vi "rqcAlice PM Level Test (Low Level Example).vi"() -> ()   [LabVIEW 2018]
uses:
  FPGA/Alice/Custom Controls/Main State Machine/rqcAlice DAC Clock Positions.ctl
  Shared/Shared FPGA Lib/Shared Logic/Custom Controls/rqc Random Generator.parameters.ctl
  Shared/Shared FPGA Lib/Shared Logic/Custom Controls/rqc Random Generator.value type.ctl
  FPGA/Alice/Custom Controls/Phase Modulator/rqcAlice Mod.Config.ctl
  Custom Controls/rqcAlice States.ctl
  Shared/Shared Host Lib/rqc ServiceNET/Custom Controls/rqc ServiceNET command.ctl
  Shared/Shared Host Lib/rqc ServiceNET/Alice/Custom Controls/rqcAlice ServiceNET control.ctl
  <vilib>/FPGAPlugInAG/PCI-7811R/niLvFpga_Open_PCI-7811R.vi
  <vilib>/rvi/interface/common/dynamic/niFpgaDynamicAddResources.vi
  <vilib>/FPGAPlugInAG/Dynamic/niLvFpga_Close_Dynamic.vi
  <vilib>/rvi/interface/nirviOpenFPGA/nirviOpenFPGA.xnode
  FPGA Bitfiles/rqcAlice FPGA (7811R) v 3.0.0.lvbitx
  <vilib>/rvi/interface/nirviCloseFPGA/nirviCloseFPGA.xnode
panel:
  in  "Attenuation, dB":fxp<+,7,6>
  in  "Delay Line":u32=24665
  out "XY Graph":T1(graph)={"appended array"=[0.0, 8.0, 16.0, 24.0, 32.0, 40.0, 48.0, 56.0, 64.0, 72.0, 80.0, 88.0, 96.0, 104.0, 112.0, 120.0, 128.0, 136.0, 144.0, 152.0, 160.0, 168.0, 176.0, 184.0, 192.0, 200.0, 208.0, 216.0, 224.0, 232.0, 240.0, 248.0, 256.0, 264.0, 272.0, 280.0, 288.0, 296.0, 304.0, 312.0, 320.0, 328.0, 336.0, 344.0, 352.0, 360.0, 368.0, 376.0, 384.0, 392.0, 400.0, 408.0, 416.0, 424.0, 432.0, 440.0, 448.0, 456.0, 464.0, 472.0, 480.0, 488.0, 496.0, 504.0, 512.0, 512.0], "appended array"=[4.0, 1.0, 6.0, 11.0, 18.0, 22.0, 32.0, 57.0, 67.0, 85.0, 91.0, 122.0, 128.0, 130.0, 145.0, 171.0, 185.0, 166.0, 196.0, 178.0, 195.0, 205.0, 197.0, 198.0, 189.0, 183.0, 188.0, 184.0, 164.0, 143.0, 127.0, 129.0, 123.0, 108.0, 77.0, 63.0, 51.0, 62.0, 40.0, 26.0, 19.0, 17.0, 19.0, 26.0, 15.0, 21.0, 28.0, 23.0, 40.0, 36.0, 69.0, 61.0, 58.0, 96.0, 93.0, 110.0, 128.0, 93.0, 112.0, 128.0, 125.0, 144.0, 161.0, 159.0, 158.0]}
  out "PM Value":u16=512
  in  "PM Delta":u16=8
  in  "PM max":u16=512
  in  "PM min":u16
  out "error out":errorcluster
  in  "Stop":bool
  out "connected?":bool
  in  "port":u16=5020
  out "Current State":T2=enum."App.Stop"
  in  "Modulator config":T3={"mod.on"=9, "mod.off"=2}
  in  "PM.DAC parameters":T4={"value type"=enum."constant", "constant"=512, "num of levels"=0, "levels values"=[512, 512, 512, 512]}
  in  "DAC Clock positions":T6=[18, 38]
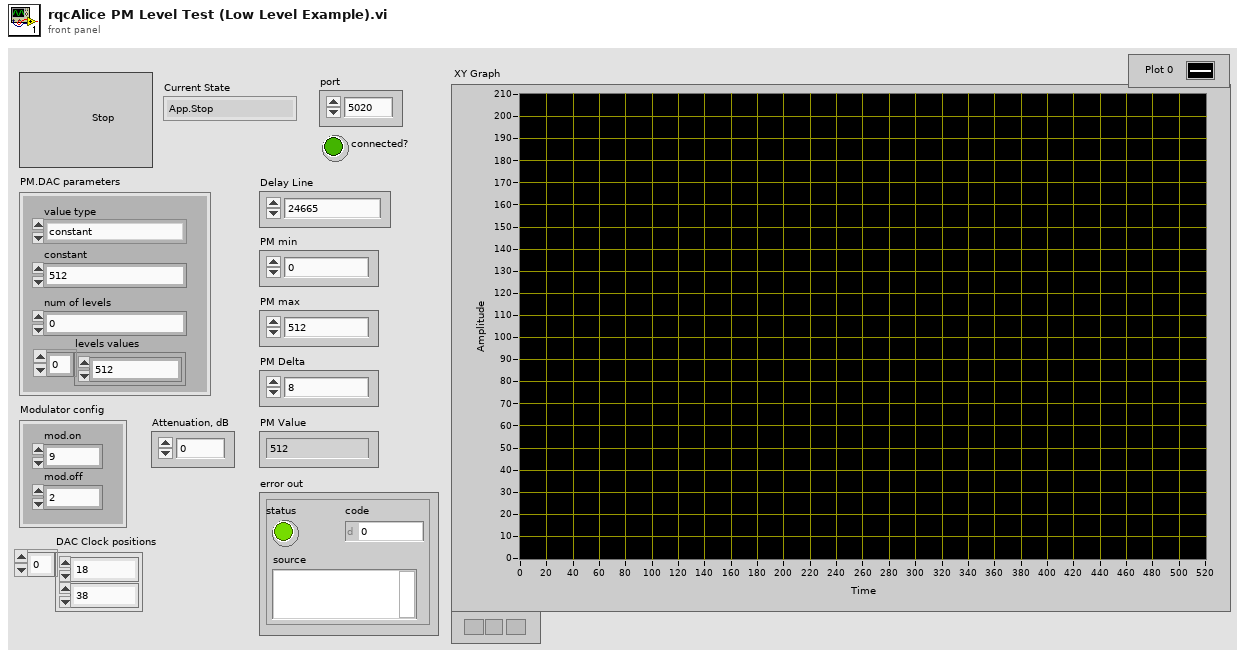
[diagram p1: front panel]
types:
  T1 = cluster{"appended array":dbl[], "appended array":dbl[]}
  T2 = typedef "rqcAlice States.ctl" = enum16{"HW.configure", "HW.meas", "NET.create", "NET.connect", "NET.readCommand", "NET.sendCommand", "NET.readData", "NET.close", "Meas.Start", "Meas.NextStep", "Meas.restart", "Meas.Done", "App.HandleEvent", "App.HandleError", "App.Stop"}
  T3 = typedef "rqcAlice Mod.Config.ctl" = cluster{"mod.on":u8, "mod.off":u8}
  T4 = typedef "rqc Random Generator.parameters.ctl" = cluster{"value type":T5, "constant":u16, "num of levels":u16, "levels values":u16[]}
  T5 = typedef "rqc Random Generator.value type.ctl" = enum16{"random value", "constant"}
  T6 = typedef "rqcAlice DAC Clock Positions.ctl" = u8[]
  T7 = typedef "rqc ServiceNET command.ctl" = enum8{"NONE", "READY", "START", "PING"}
  T8 = typedef "rqcAlice ServiceNET control.ctl" = cluster{"connection ID":refnum<k5>, "port":u16, "connected?":bool}
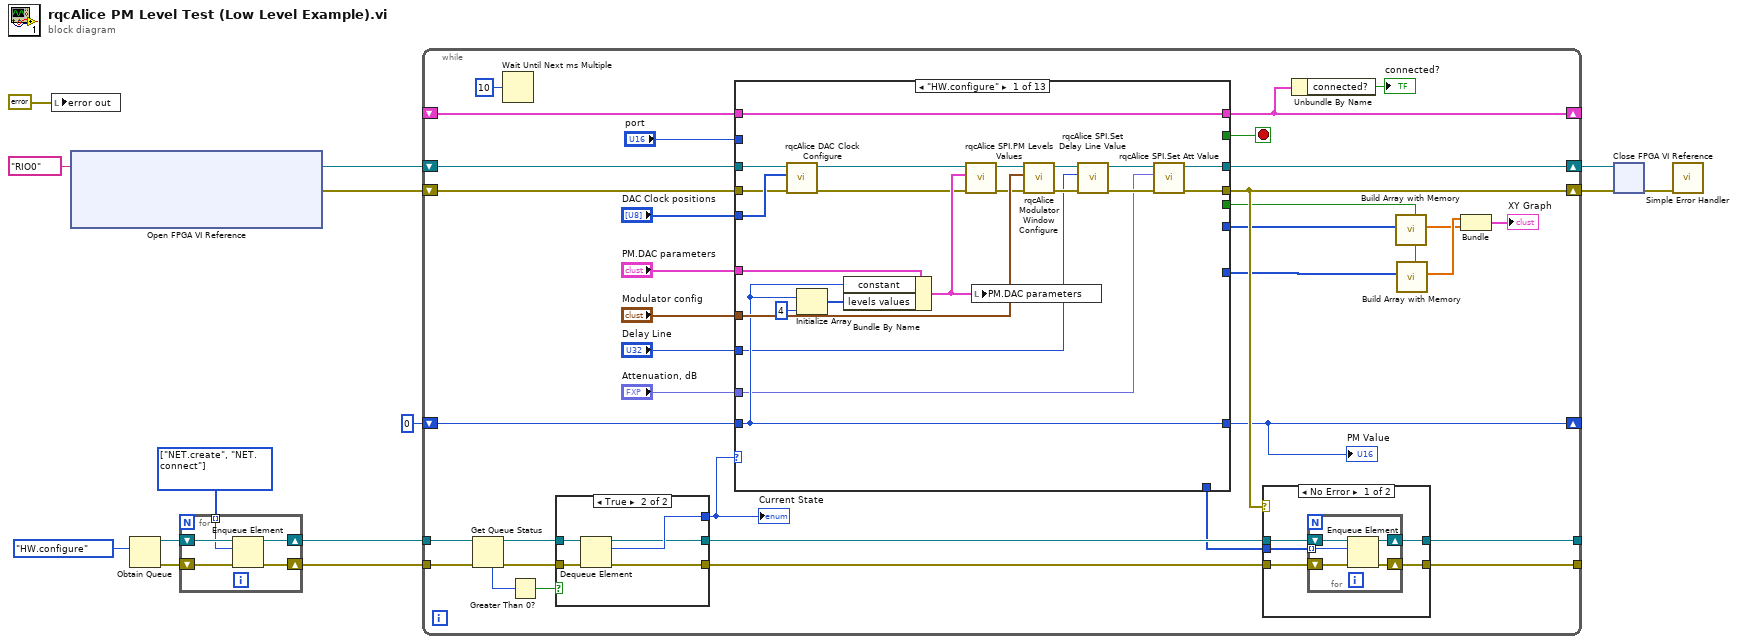
[diagram p0: block diagram]
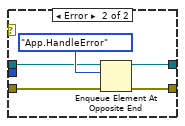
[diagram p2: hidden frame]
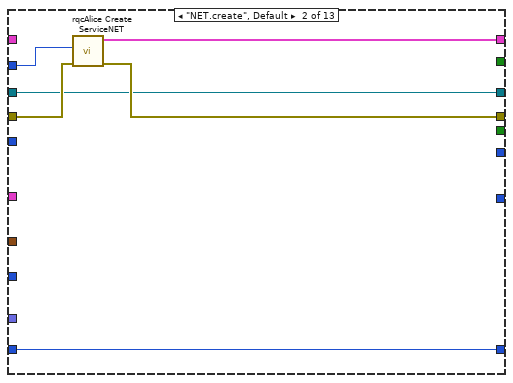
[diagram p3: hidden frame]
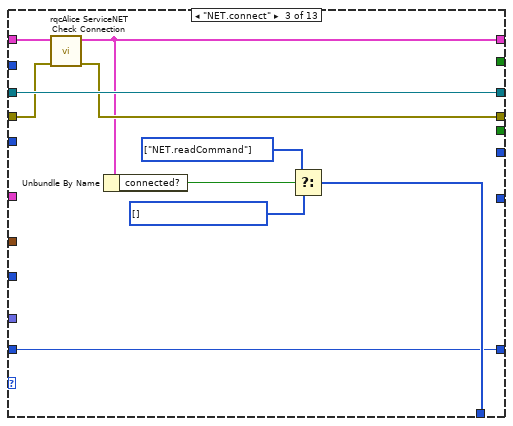
[diagram p4: hidden frame]
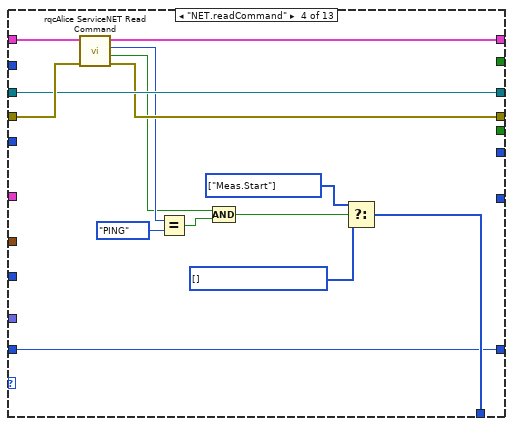
[diagram p5: hidden frame]
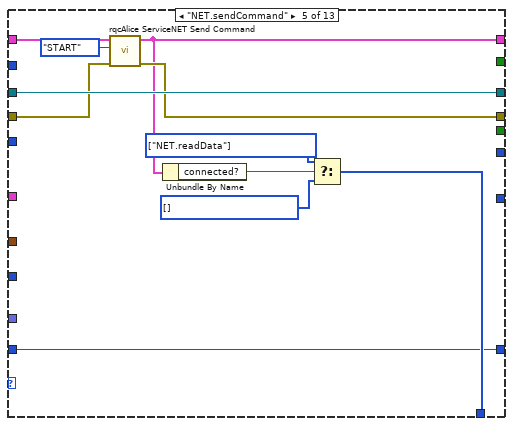
[diagram p6: hidden frame]
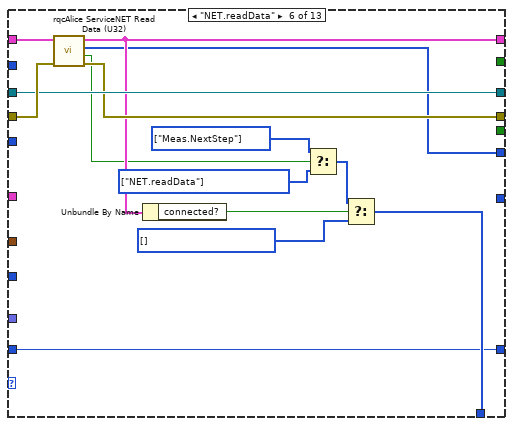
[diagram p7: hidden frame]
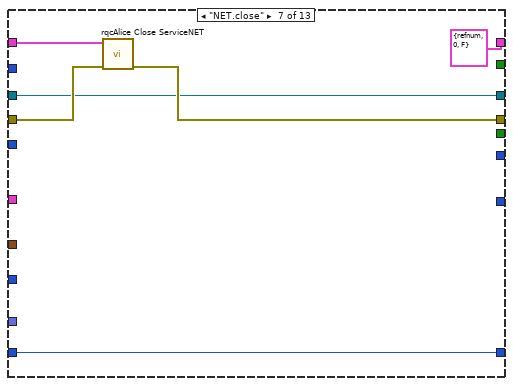
[diagram p8: hidden frame]
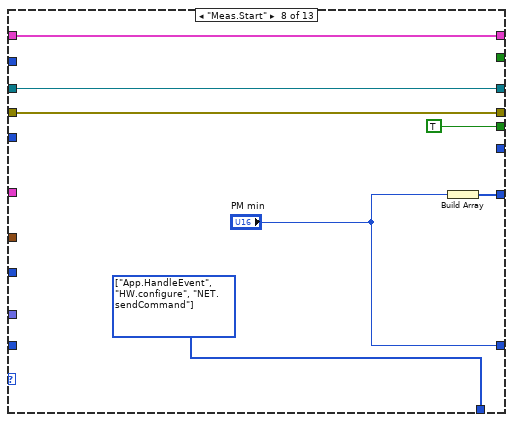
[diagram p9: hidden frame]
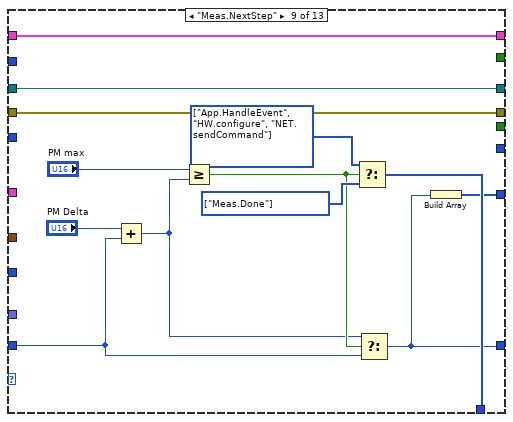
[diagram p10: hidden frame]
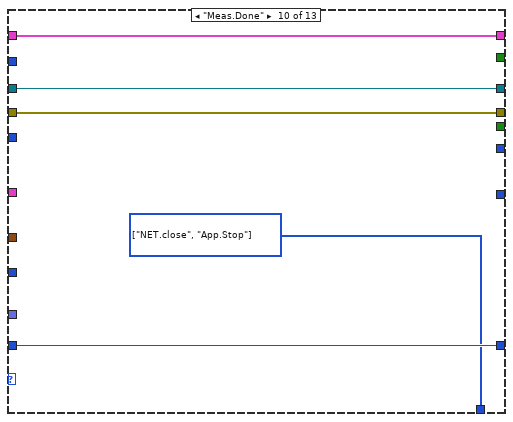
[diagram p11: hidden frame]
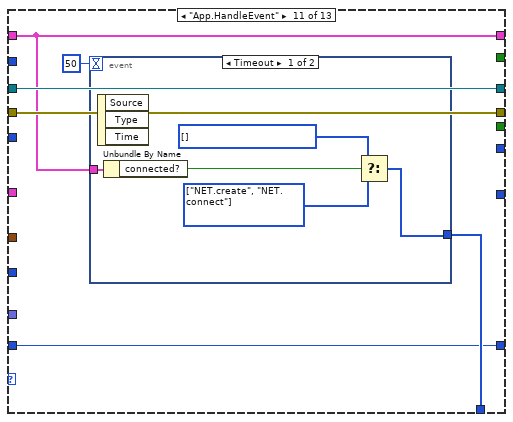
[diagram p12: hidden frame]
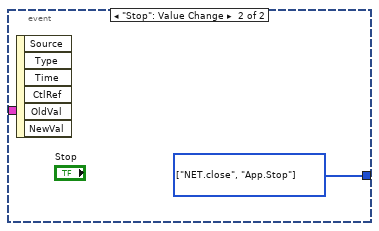
[diagram p13: hidden frame]
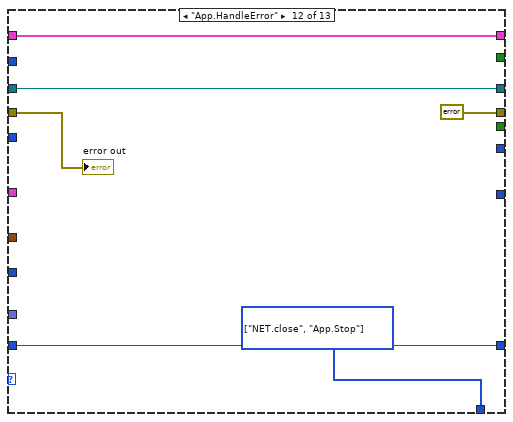
[diagram p14: hidden frame]
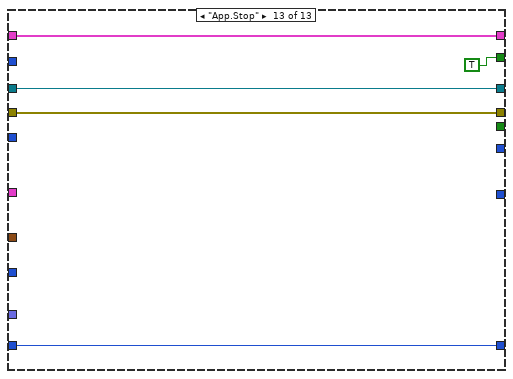
[diagram p15: hidden frame]
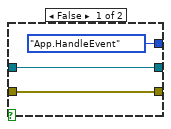
[diagram p16: hidden frame]
diagram:
  w6 = T2[] [enum."NET.create", enum."NET.connect"] items=["HW.configure", "HW.meas", "NET.create", "NET.connect", "NET.readCommand", "NET.sendCommand", "NET.readData", "NET.close", "Meas.Start", "Meas.NextStep", "Meas.restart", "Meas.Done", "App.HandleEvent", "App.HandleError", "App.Stop"]
  n1 = local write "error out"(errorcluster {"status"=FALSE, "code"=0, "source"=""} ("error out")) -> ()
  n2 = xnode "Open FPGA VI Reference"("resource name"=tag "RIO0") -> ("FPGA VI Reference Out"=w13:refnum<k20>, "error out"=w12:errorcluster)  [unwired: 1 in]
  n3 = Obtain Queue(element data type=rqcAlice_States."HW.configure" ("rqcAlice States")) -> (queue out=w8:refnum<queue>, error out=w7:errorcluster)  [unwired: 4 in, 1 out]
  n4 = for {
    shift-right: [w17] -> w5
    shift-left: w8 -> [w19]
    shift-right: [w16] -> w4
    shift-left: w7 -> [w18]
    tunnel: w6 -> [w15] mode=indexing
    n5 = Enqueue Element(queue=w19, element=w15, error in (no error)=w18) -> (queue out=w17:refnum<queue>, error out=w16:errorcluster)  [unwired: 1 in, 1 out]
  }
  n6 = while {
    tunnel: w5 -> [w48]
    shift-right: [w49] -> w11
    shift-left: w13 -> [w54]
    shift-right: [w41] -> w10
    shift-left: w12 -> [w52]
    tunnel: w4 -> [w47]
    tunnel: [w38] -> _
    tunnel: [w37] -> _
    shift-right: [w33] -> _
    shift-left: _ -> [w35]
    shift-right: [w27] -> _
    shift-left: u16 0 ("Delay Line min") -> [w29]
    stop <- w31 stop-if-true
    n7 = Get Queue Status(queue=w48, error in (no error)=w47) -> (queue out=w44:refnum<queue>, error out=w43:errorcluster, # elements in queue=w46:i32)  [unwired: 1 in, 5 out]
    n8 = Wait Until Next ms Multiple(millisecond multiple=u32 10) -> ()  [unwired: 1 out]
    n9 = Greater Than 0?(x=w46) -> (x > 0?=w45:bool)
    n10 = case shown="True" w45 {
      tunnel: w44 -> [w202 w208]
      tunnel: w43 -> [w201 w207]
      tunnel: [rqcAlice_States."App.HandleEvent" ("rqcAlice States") w206] -> w42
      tunnel: [w202 w205] -> w40
      tunnel: [w201 w204] -> w39
      frame False {
      }
      frame True {
        n11 = Dequeue Element(queue=w208, error in (no error)=w207) -> (queue out=w205:refnum<queue>, element=w206:T2, error out=w204:errorcluster)  [unwired: 1 in, 1 out]
      }
    }
    "Current State" <- w42
    n12 = case shown="\"HW.configure\"" w42 {
      tunnel: w54 -> [w91 w94 w107 w118 w132 w144 w148 w158 w171 w176 w183 w194 w199]
      tunnel: "DAC Clock positions" -> [w90 _ _ _ _ _ _ _ _ _ _ _ _]
      tunnel: w52 -> [w89 w96 w105 w120 w130 w145 w151 w157 w170 w175 w182 w193 w198]
      tunnel: "PM.DAC parameters" -> [w86 _ _ _ _ _ _ _ _ _ _ _ _]
      tunnel: "Modulator config" -> [w88 _ _ _ _ _ _ _ _ _ _ _ _]
      tunnel: [w78 w94 w107 w118 w132 w144 w148 w158 w171 w176 w183 w194 w199] -> w49
      tunnel: [w76 w95 w104 w117 w129 w143 w150 w157 w170 w175 w182 errorcluster {"status"=FALSE, "code"=0, "source"=""} ("error out") w198] -> w41
      tunnel: [_ _ w100 w109 w123 w135 _ w156 w166 w173 w179 w191 _] -> w36
      tunnel: [w87 w97 w103 w119 w127 w142 T8 {"connection ID"=refnum, "port"=0, "connected?"=FALSE} ("rqcAlice ServiceNET out") w159 w172 w177 w180 w195 w197] -> w33
      tunnel: w35 -> [w87 _ w106 w121 w131 w146 w152 w159 w172 w177 w180 w195 w197]
      tunnel: "port" -> [_ w93 _ _ _ _ _ _ _ _ _ _ _]
      tunnel: [_ _ _ _ _ _ _ _ _ _ _ _ TRUE] -> w31
      tunnel: w29 -> [w83 w92 w98 w108 w122 w134 w147 _ w162 w174 w178 w190 w196]
      tunnel: [w83 w92 w98 w108 w122 w134 w147 "PM min" w161 w174 w178 w190 w196] -> w27
      tunnel: [_ _ _ _ _ w133 _ _ _ _ _ _ _] -> w28
      tunnel: [_ _ _ _ _ _ _ w153 w160 _ _ _ _] -> w26
      tunnel: [_ _ _ _ _ _ _ TRUE _ _ _ _ _] -> w25
      tunnel: "Delay Line" -> [w80 _ _ _ _ _ _ _ _ _ _ _ _]
      tunnel: "Attenuation, dB" -> [w75 _ _ _ _ _ _ _ _ _ _ _ _]
      frame "HW.configure" {
        n13 = call "rqcAlice DAC Clock Configure.vi"("error in"=w89, "DAC Clock params"=w90, "Alice FPGA Reference In"=w91) -> ("error out"=w72:errorcluster, "Alice FPGA Reference Out"=w74:refnum<k20>)  [unwired: 7 in]
        n14 = Initialize Array(w83, 4 ("dimension size")) -> (w84:u16[])
        n15 = Bundle By Name(cluster=w86, "constant"=w83, "levels values"=w84) -> (w73:T4)
        n16 = call "rqcAlice SPI.PM Levels Values.vi"("error in"=w72, "RndGen.parameters"=w73, "Alice FPGA Reference In"=w74) -> ("error out"=w71:errorcluster, "Alice FPGA Reference Out"=w70:refnum<k20>)  [unwired: 6 in, 1 out]
        n17 = local write "PM.DAC parameters"(w73) -> ()
        n18 = call "rqcAlice Modulator Window Configure.vi"("error in"=w71, "Modulator config"=w88, "Alice FPGA Reference In"=w70) -> ("error out"=w82:errorcluster, "Alice FPGA Reference Out"=w81:refnum<k20>)  [unwired: 7 in]
        n19 = call "rqcAlice SPI.Set Delay Line Value.vi"("error in"=w82, "Delay Line Value"=w80, "Alice FPGA Reference In"=w81) -> ("error out"=w77:errorcluster, "Alice FPGA Reference Out"=w79:refnum<k20>)  [unwired: 7 in]
        n20 = call "rqcAlice SPI.Set Att Value.vi"("error in"=w77, "Attenuation, dB"=w75, "Alice FPGA Reference In"=w79) -> ("error out"=w76:errorcluster, "Alice FPGA Reference Out"=w78:refnum<k20>)  [unwired: 7 in]
      }
      frame "NET.create", Default {
        n21 = call "rqcAlice Create ServiceNET.vi"("error in"=w96, "port"=w93) -> ("error out"=w95:errorcluster, "rqcAlice ServiceNET control"=w97:T8)  [unwired: 8 in]
      }
      frame "NET.connect" {
        w99 = T2[] [] items=["HW.configure", "HW.meas", "NET.create", "NET.connect", "NET.readCommand", "NET.sendCommand", "NET.readData", "NET.close", "Meas.Start", "Meas.NextStep", "Meas.restart", "Meas.Done", "App.HandleEvent", "App.HandleError", "App.Stop"] ("f")
        w101 = T2[] [enum."NET.readCommand"] items=["HW.configure", "HW.meas", "NET.create", "NET.connect", "NET.readCommand", "NET.sendCommand", "NET.readData", "NET.close", "Meas.Start", "Meas.NextStep", "Meas.restart", "Meas.Done", "App.HandleEvent", "App.HandleError", "App.Stop"]
        n22 = call "rqcAlice ServiceNET Check Connection.vi"("error in"=w105, "rqcAlice ServiceNET in"=w106) -> ("error out"=w104:errorcluster, "rqcAlice ServiceNET out"=w103:T8)  [unwired: 8 in]
        n23 = Unbundle By Name(w103) -> ("connected?"=w102:bool)
        n24 = Select(t=w101, s=w102, f=w99) -> (s? t:f=w100:T2[])
      }
      frame "NET.readCommand" {
        w110 = T2[] [] items=["HW.configure", "HW.meas", "NET.create", "NET.connect", "NET.readCommand", "NET.sendCommand", "NET.readData", "NET.close", "Meas.Start", "Meas.NextStep", "Meas.restart", "Meas.Done", "App.HandleEvent", "App.HandleError", "App.Stop"] ("f")
        w111 = T2[] [enum."Meas.Start"] items=["HW.configure", "HW.meas", "NET.create", "NET.connect", "NET.readCommand", "NET.sendCommand", "NET.readData", "NET.close", "Meas.Start", "Meas.NextStep", "Meas.restart", "Meas.Done", "App.HandleEvent", "App.HandleError", "App.Stop"] ("f")
        n25 = call "rqcAlice ServiceNET Read Command.vi"("error in"=w120, "rqcAlice ServiceNET in"=w121) -> ("error out"=w117:errorcluster, "cmd valid"=w113:bool, "command"=w115:T7, "rqcAlice ServiceNET out"=w119:T8)  [unwired: 6 in]
        n26 = Equal?(x=w115, y=rqc_ServiceNET_command."PING" ("command")) -> (x = y?=w114:bool)
        n27 = Compound Arithmetic op=AND(w113, w114) -> (w112:bool)
        n28 = Select(t=w111, s=w112, f=w110) -> (s? t:f=w109:T2[])
      }
      frame "NET.sendCommand" {
        w124 = T2[] [] items=["HW.configure", "HW.meas", "NET.create", "NET.connect", "NET.readCommand", "NET.sendCommand", "NET.readData", "NET.close", "Meas.Start", "Meas.NextStep", "Meas.restart", "Meas.Done", "App.HandleEvent", "App.HandleError", "App.Stop"] ("f")
        w125 = T2[] [enum."NET.readData"] items=["HW.configure", "HW.meas", "NET.create", "NET.connect", "NET.readCommand", "NET.sendCommand", "NET.readData", "NET.close", "Meas.Start", "Meas.NextStep", "Meas.restart", "Meas.Done", "App.HandleEvent", "App.HandleError", "App.Stop"] ("f")
        n29 = call "rqcAlice ServiceNET Send Command.vi"("error in"=w130, "command"=rqc_ServiceNET_command."START", "rqcAlice ServiceNET in"=w131) -> ("error out"=w129:errorcluster, "rqcAlice ServiceNET out"=w127:T8)  [unwired: 7 in]
        n30 = Unbundle By Name(w127) -> ("connected?"=w126:bool)
        n31 = Select(t=w125, s=w126, f=w124) -> (s? t:f=w123:T2[])
      }
      frame "NET.readData" {
        w136 = T2[] [] items=["HW.configure", "HW.meas", "NET.create", "NET.connect", "NET.readCommand", "NET.sendCommand", "NET.readData", "NET.close", "Meas.Start", "Meas.NextStep", "Meas.restart", "Meas.Done", "App.HandleEvent", "App.HandleError", "App.Stop"] ("f")
        w141 = T2[] [enum."Meas.NextStep"] items=["HW.configure", "HW.meas", "NET.create", "NET.connect", "NET.readCommand", "NET.sendCommand", "NET.readData", "NET.close", "Meas.Start", "Meas.NextStep", "Meas.restart", "Meas.Done", "App.HandleEvent", "App.HandleError", "App.Stop"] ("t")
        w139 = T2[] [enum."NET.readData"] items=["HW.configure", "HW.meas", "NET.create", "NET.connect", "NET.readCommand", "NET.sendCommand", "NET.readData", "NET.close", "Meas.Start", "Meas.NextStep", "Meas.restart", "Meas.Done", "App.HandleEvent", "App.HandleError", "App.Stop"] ("f")
        n32 = call "rqcAlice ServiceNET Read Data (U32).vi"("error in"=w145, "rqcAlice ServiceNET in"=w146) -> ("error out"=w143:errorcluster, "data valid"=w140:bool, "data"=w133:u32[], "rqcAlice ServiceNET out"=w142:T8)  [unwired: 6 in]
        n33 = Unbundle By Name(w142) -> ("connected?"=w138:bool)
        n34 = Select(t=w141, s=w140, f=w139) -> (s? t:f=w137:T2[])
        n35 = Select(t=w137, s=w138, f=w136) -> (s? t:f=w135:T2[])
      }
      frame "NET.close" {
        n36 = call "rqcAlice Close ServiceNET.vi"("error in"=w151, "rqcAlice ServiceNET in"=w152) -> ("error out"=w150:errorcluster)  [unwired: 9 in]
      }
      frame "Meas.Start" {
        w156 = T2[] [enum."App.HandleEvent", enum."HW.configure", enum."NET.sendCommand"] items=["HW.configure", "HW.meas", "NET.create", "NET.connect", "NET.readCommand", "NET.sendCommand", "NET.readData", "NET.close", "Meas.Start", "Meas.NextStep", "Meas.restart", "Meas.Done", "App.HandleEvent", "App.HandleError", "App.Stop"] ("f")
        n37 = Build Array("PM min") -> (w153:u16[])
      }
      frame "Meas.NextStep" {
        w165 = T2[] [enum."Meas.Done"] items=["HW.configure", "HW.meas", "NET.create", "NET.connect", "NET.readCommand", "NET.sendCommand", "NET.readData", "NET.close", "Meas.Start", "Meas.NextStep", "Meas.restart", "Meas.Done", "App.HandleEvent", "App.HandleError", "App.Stop"] ("f")
        w167 = T2[] [enum."App.HandleEvent", enum."HW.configure", enum."NET.sendCommand"] items=["HW.configure", "HW.meas", "NET.create", "NET.connect", "NET.readCommand", "NET.sendCommand", "NET.readData", "NET.close", "Meas.Start", "Meas.NextStep", "Meas.restart", "Meas.Done", "App.HandleEvent", "App.HandleError", "App.Stop"] ("f")
        n38 = Add(x="PM Delta", y=w162) -> (x+y=w163:u16)
        n39 = Greater Or Equal?(x="PM max", y=w163) -> (x >= y?=w164:bool)
        n40 = Select(t=w167, s=w164, f=w165) -> (s? t:f=w166:T2[])
        n41 = Select(t=w163, s=w164, f=w162) -> (s? t:f=w161:u16)
        n42 = Build Array(w161) -> (w160:u16[])
      }
      frame "Meas.Done" {
        w173 = T2[] [enum."NET.close", enum."App.Stop"] items=["HW.configure", "HW.meas", "NET.create", "NET.connect", "NET.readCommand", "NET.sendCommand", "NET.readData", "NET.close", "Meas.Start", "Meas.NextStep", "Meas.restart", "Meas.Done", "App.HandleEvent", "App.HandleError", "App.Stop"] ("f")
      }
      frame "App.HandleEvent" {
        n43 = event shown="[0] Timeout" {
          selector: _ -> [_ _]
          dyn-events: _ -> [_ _]
          timeout: 50 -> [_ _]
          tunnel: w180 -> [w188 _]
          tunnel: [w184 w189] -> w179
          event Timeout {
            w185 = T2[] [enum."NET.create", enum."NET.connect"] items=["HW.configure", "HW.meas", "NET.create", "NET.connect", "NET.readCommand", "NET.sendCommand", "NET.readData", "NET.close", "Meas.Start", "Meas.NextStep", "Meas.restart", "Meas.Done", "App.HandleEvent", "App.HandleError", "App.Stop"]
            w186 = T2[] [] items=["HW.configure", "HW.meas", "NET.create", "NET.connect", "NET.readCommand", "NET.sendCommand", "NET.readData", "NET.close", "Meas.Start", "Meas.NextStep", "Meas.restart", "Meas.Done", "App.HandleEvent", "App.HandleError", "App.Stop"]
            n44 = event-data() -> ()  [unwired: 1 in, 3 out]
            n45 = Unbundle By Name(w188) -> ("connected?"=w187:bool)
            n46 = Select(t=w186, s=w187, f=w185) -> (s? t:f=w184:T2[])
          }
          event "Stop": Value Change {
            w189 = T2[] [enum."NET.close", enum."App.Stop"] items=["HW.configure", "HW.meas", "NET.create", "NET.connect", "NET.readCommand", "NET.sendCommand", "NET.readData", "NET.close", "Meas.Start", "Meas.NextStep", "Meas.restart", "Meas.Done", "App.HandleEvent", "App.HandleError", "App.Stop"]
            n47 = event-data() -> ()  [unwired: 1 in, 6 out]
          }
        }
      }
      frame "App.HandleError" {
        w191 = T2[] [enum."NET.close", enum."App.Stop"] items=["HW.configure", "HW.meas", "NET.create", "NET.connect", "NET.readCommand", "NET.sendCommand", "NET.readData", "NET.close", "Meas.Start", "Meas.NextStep", "Meas.restart", "Meas.Done", "App.HandleEvent", "App.HandleError", "App.Stop"] ("f")
        "error out" <- w193
      }
      frame "App.Stop" {
      }
    }
    "PM Value" <- w27
    n48 = case shown="No Error" w41 {
      tunnel: w40 -> [w59 w68]
      tunnel: w39 -> [w58 w66]
      tunnel: [w57 w67] -> w38
      tunnel: [w56 w65] -> w37
      tunnel: w36 -> [w55 _]
      frame No Error {
        n49 = for {
          shift-right: [w62] -> w57
          shift-left: w59 -> [w64]
          shift-right: [w61] -> w56
          shift-left: w58 -> [w63]
          tunnel: w55 -> [w60] mode=indexing
          n50 = Enqueue Element(queue=w64, element=w60, error in (no error)=w63) -> (queue out=w62:refnum<queue>, error out=w61:errorcluster)  [unwired: 1 in, 1 out]
        }
      }
      frame Error {
        n51 = Enqueue Element At Opposite End(queue=w68, element=rqcAlice_States."App.HandleError" ("rqcAlice States"), error in (no error)=w66) -> (queue out=w67:refnum<queue>, error out=w65:errorcluster)  [unwired: 1 in, 1 out]
      }
    }
    n52 = Unbundle By Name(w33) -> ("connected?"=→"connected?":bool)
    n53 = call "Build Array with Memory.vi"("reset"=w25, "new array"=w28) -> ("appended array"=w22:dbl[])  [unwired: 9 in]
    n54 = call "Build Array with Memory.vi"("reset"=w25, "new array"=w26) -> ("appended array"=w23:dbl[])  [unwired: 9 in]
    n55 = Bundle("appended array"=w23, "appended array"=w22) -> (→"XY Graph":T1)  [unwired: 1 in]
  }
  n56 = xnode "Close FPGA VI Reference"("FPGA VI Reference In"=w11, "error in"=w10) -> ("error out"=w3:errorcluster)
  n57 = call <vilib>:"Simple Error Handler.vi"("error in (no error)"=w3) -> ()  [unwired: 4 in, 5 out]
